vi "Response Error.vi"(8 "error in (no error)":errorcluster, 10 "Message":string, 11 "Name":string) -> (0 "error out":errorcluster, 2 "last notification":errorcluster)   [LabVIEW 2019, in "Error Notifier.lvlib"]
uses:
  Error Notifier.lvlib
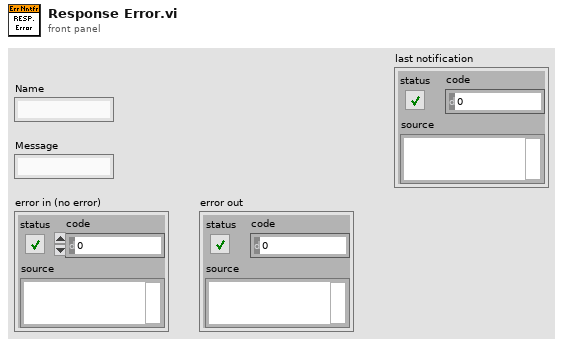
[diagram p1: front panel]
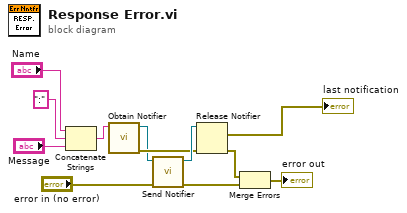
[diagram p0: block diagram]
diagram:
  n1 = Concatenate Strings("Name", ":" ("string"), "Message") -> (w2:string)
  n2 = call "Obtain Notifier.vi"("Name"=w2) -> ("Error Out"=w8:errorcluster, "notifier out"=w6:refnum<notifier>)  [unwired: 9 in]
  n3 = call "Send Notifier.vi"("Error In"="error in (no error)", "notifier in"=w6) -> ("Error Out"=w12:errorcluster, "notifier out"=w9:refnum<notifier>)  [unwired: 8 in]
  n4 = Release Notifier(notifier=w9, error in (no error)=w8) -> (last notification=→"last notification":errorcluster, error out=w11:errorcluster)  [unwired: 1 in, 1 out]
  n5 = Merge Errors(w11, w12) -> (→"error out":errorcluster)
